vi "Receive command.vi"(8 "error in (no error)":errorcluster) -> (0 "error out":errorcluster, 2 "Data":variant, 3 "command":string)   [LabVIEW 2020, in "queue_core_loop.lvlib"]
uses:
  queue_core_loop.lvlib
panel:
  # "Development\ncontrols/indicators useful for development and testing, but which are not outputs of the VI"
  # "Input\nInputs to the VI"
  # "Output\nOutputs of the VI"
  # "Description\n\nBlank VI with error handling case. \n\nSummarize the use of this VI in this space."
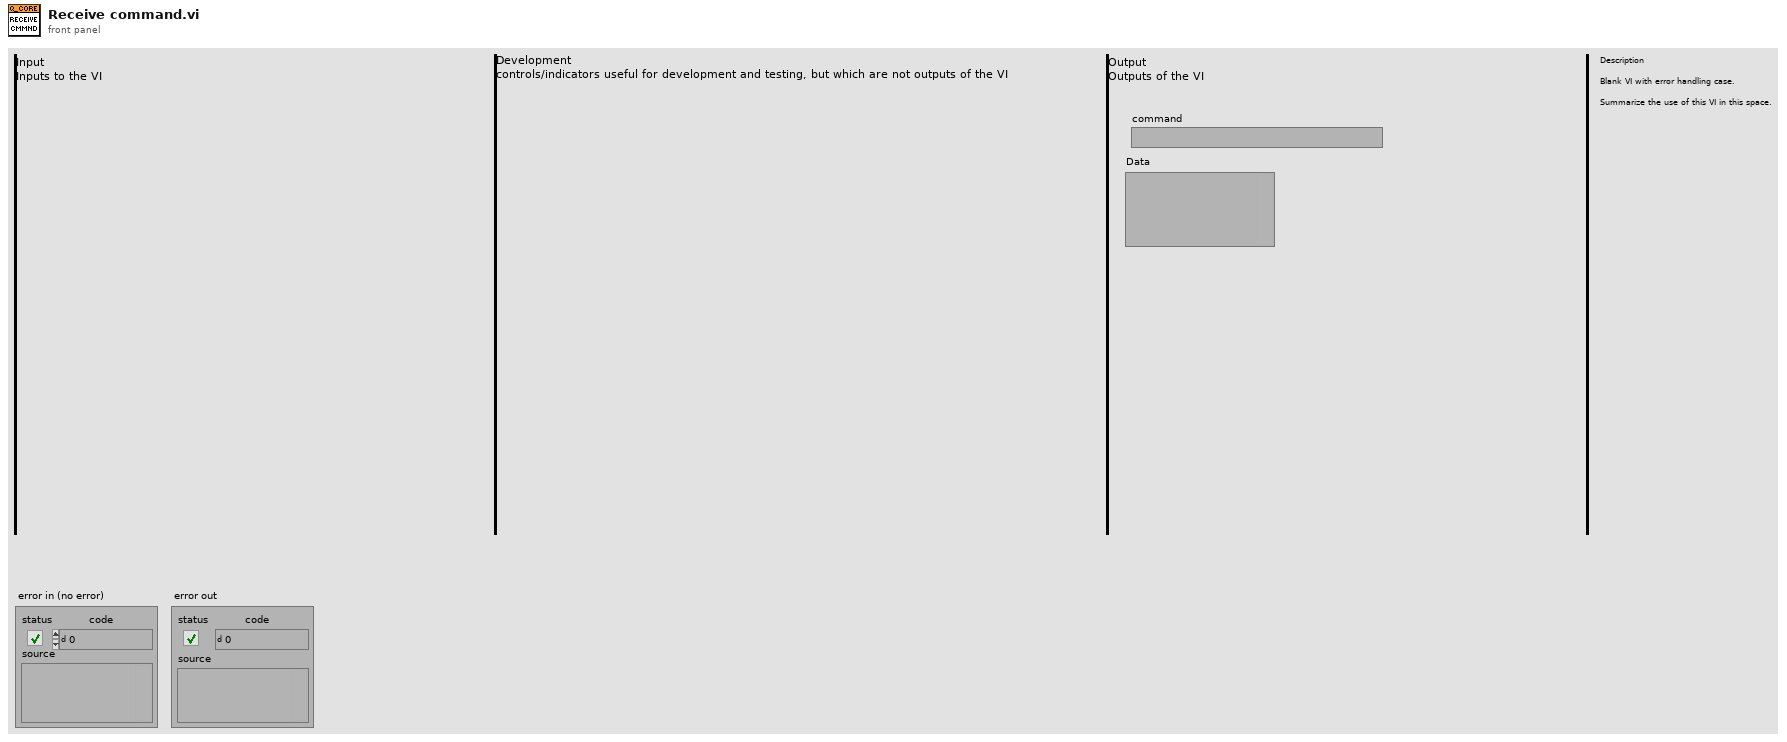
[diagram p1: front panel]
types:
  T1 = typedef "dev_and_debug_tools.lvlib/QueueMessage typedef.ctl" = cluster{"command":string, "data":variant}
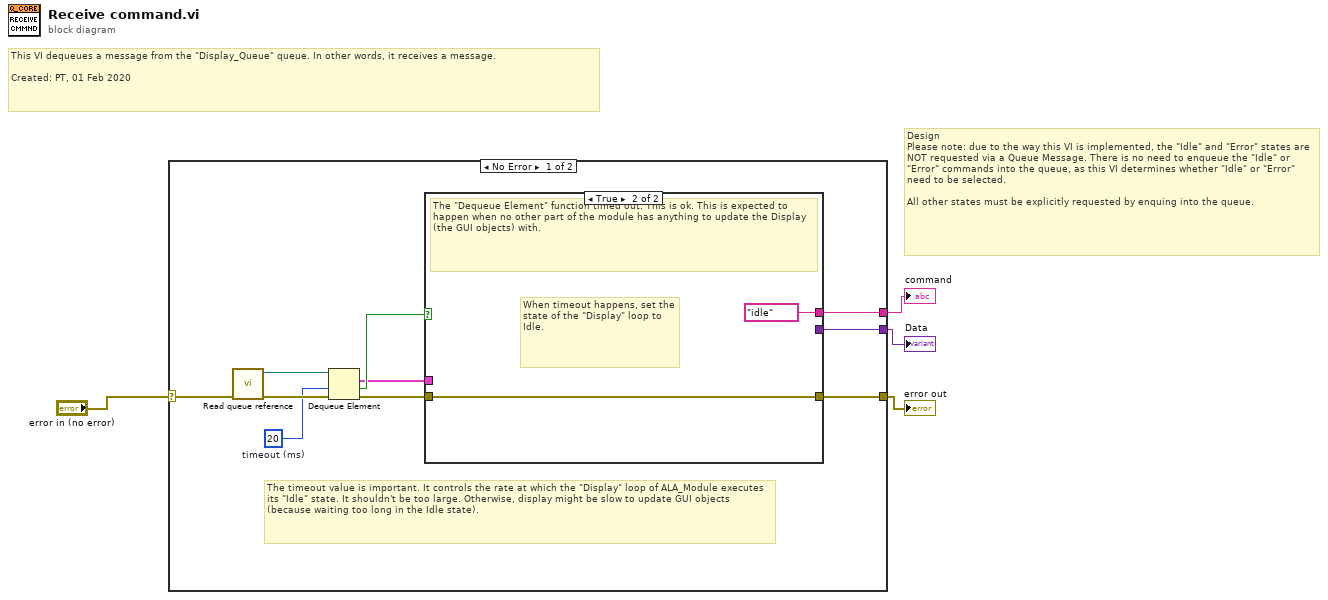
[diagram p0: block diagram]
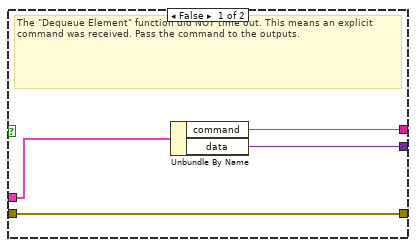
[diagram p2: hidden frame]
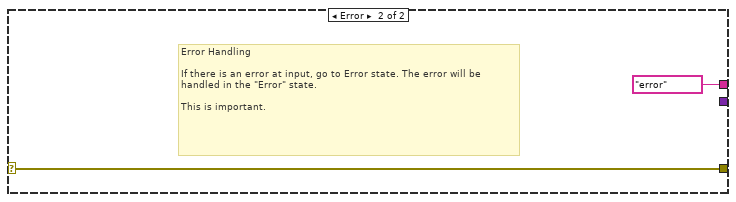
[diagram p3: hidden frame]
diagram:
  # "Design\nPlease note: due to the way this VI is implemented, the \"Idle\" and \"Error\" states are NOT requested via a Queue Message. There is no need to enqueue the \"Idle\" or \"Error\" commands into the queue, as this VI determines whether \"Idle\" or \"Error\" need to be selected.\n\nAll other states must be explicitly requested by enquing into the queue."
  # "This VI dequeues a message from the \"Display_Queue\" queue. In other words, it receives a message.\n\nCreated: PT, 01 Feb 2020"
  n1 = case shown="No Error" "error in (no error)" {
    selector: "error in (no error)" -> [w14 w22]
    tunnel: [w7 w22] -> w3
    tunnel: [w6 _] -> w2
    tunnel: [w5 "error" ("command")] -> w1
    frame No Error {
      w11 = 20  # timeout (ms)
      # "The timeout value is important. It controls the rate at which the \"Display\" loop of ALA_Module executes its \"Idle\" state. It shouldn't be too large. Otherwise, display might be slow to update GUI objects (because waiting too long in the Idle state)."
      n2 = call "Read queue reference.vi"("error in (no error)"=w14) -> ("error out"=w13:errorcluster, "ALA_Display_Queue ref"=w12:refnum<queue>)  [unwired: 9 in]
      n3 = Dequeue Element(queue=w12, timeout in ms (-1)=w11, error in (no error)=w13) -> (element=w8:T1, timed out?=w10:bool, error out=w9:errorcluster)  [unwired: 1 out]
      n4 = case shown="True" w10 {
        tunnel: w9 -> [w18 w20]
        tunnel: w8 -> [w17 _]
        tunnel: [w18 w20] -> w7
        tunnel: [w16 _] -> w6
        tunnel: [w15 "idle" ("command")] -> w5
        frame False {
          # "The \"Dequeue Element\" function did NOT time out. This means an explicit command was received. Pass the command to the outputs."
          n5 = Unbundle By Name(w17) -> ("command"=w15:string, "data"=w16:variant)
        }
        frame True {
          # "When timeout happens, set the state of the \"Display\" loop to Idle."
          # "The \"Dequeue Element\" function timed out. This is ok. This is expected to happen when no other part of the module has anything to update the Display (the GUI objects) with."
        }
      }
    }
    frame Error {
      # "Error Handling\n\nIf there is an error at input, go to Error state. The error will be handled in the \"Error\" state.\n\nThis is important."
    }
  }
  "error out" <- w3
  "Data" <- w2
  "command" <- w1
